vi "EvaluateBurstTriggers.vi"(8 "error in (no error)":errorcluster, 9 "data":T2, 10 "config":T1, 11 "Qbus in":refnum<class "Qbus.lvclass">) -> (0 "error out":errorcluster, 2 "config out":T1)   [LabVIEW 2017, in "BurstMode.lvlib"]
uses:
  <vilib>/addons/InsightCM/Devices/Shared/Cms/CmsBurstMode/BurstMode.lvlib
  <vilib>/addons/Qbus/Qbus.lvclass
  <vilib>/addons/InsightCM/Devices/Shared/Common/DataFlow/controls/Data.ctl
  <vilib>/addons/InsightCM/Utilities/DataAccessors/controls/wfmSGL_DVR.ctl
  <vilib>/addons/PointValueMap/controls/PointMap.ctl
  <vilib>/addons/InsightCM/Devices/Shared/Common/DataFlow/controls/Type.ctl
  <vilib>/addons/InsightCM/Devices/Shared/Cms/CmsBurstMode/controls/config.ctl
  <vilib>/addons/InsightCM/Devices/Shared/Cms/CmsBurstMode/controls/InitiateBurstMode.ctl
  <vilib>/addons/PointValueMap/PointValueMap.lvlib
  <vilib>/addons/InsightCM/Devices/Shared/Common/DataFlow/DataFlow.lvlib
panel:
  in  "force burst":bool
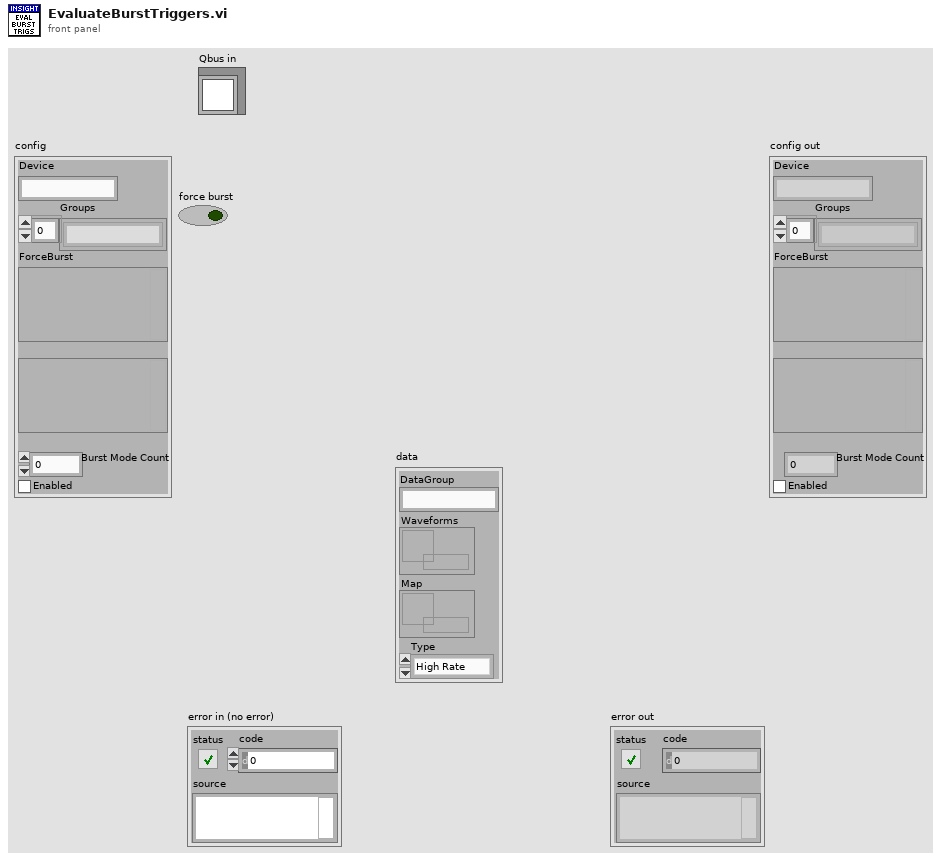
[diagram p1: front panel]
types:
  T1 = typedef "BurstMode.lvlib/config.ctl" = cluster{"Device":string, "Groups":string[], "ForceBurst":variant, "TriggerBurst":variant, "Burst Mode Count":i32, "Enabled":bool}
  T2 = typedef "DataFlow.lvlib/Data.ctl" = cluster{"DataGroup":string, "Waveforms":T3, "Map":T4, "Type":T5}
  T3 = typedef "wfmSGL_DVR.ctl" = refnum<data-value>
  T4 = typedef "PointValueMap.lvlib/PointMap.ctl" = refnum<data-value>
  T5 = typedef "DataFlow.lvlib/Type.ctl" = enum16{"High Rate", "Low Rate", "Burst Mode"}
  T6 = typedef "BurstMode.lvlib/InitiateBurstMode.ctl" = cluster{"Group":string, "Acq Reason":string}
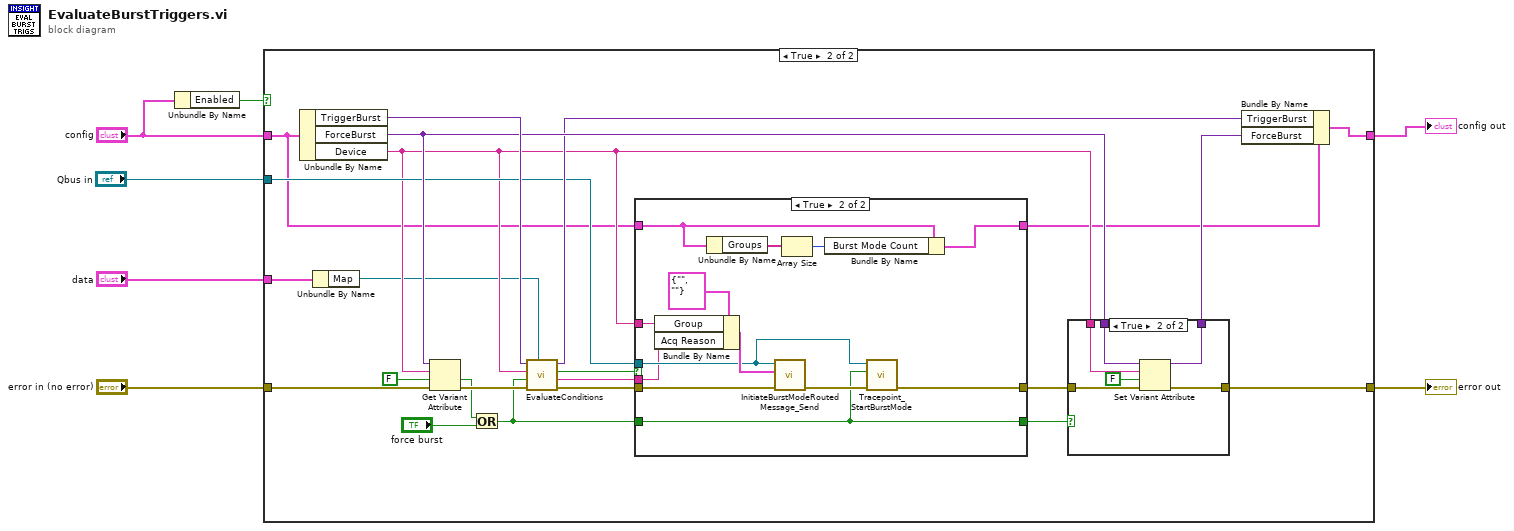
[diagram p0: block diagram]
diagram:
  n1 = Unbundle By Name("config") -> ("Enabled"=w1:bool)
  n2 = case shown="True" w1 {
    tunnel: [w8 w32] -> w7
    tunnel: "data" -> [_ w30]
    tunnel: "error in (no error)" -> [w8 w29]
    tunnel: [w9 w21] -> w4
    tunnel: "Qbus in" -> [_ w20]
    tunnel: "config" -> [w9 w13]
    frame False {
    }
    frame True {
      n3 = Unbundle By Name(w13) -> ("TriggerBurst"=w26:variant, "ForceBurst"=w25:variant, "Device"=w19:string)
      n4 = Unbundle By Name(w30) -> ("Map"=w10:T4)
      n5 = Get Variant Attribute(Variant=w25, name=w19, default value (empty Variant)=FALSE ("force trigger"), error in=w29) -> (value=w18:bool, error out=w27:errorcluster)  [unwired: 2 out]
      n6 = Or(x=w18, y="force burst") -> (x .or. y?=w16:bool)
      n7 = call <vilib>:"EvaluateConditions.vi"("map"=w10, "error in"=w27, "force burst"=w16, "device"=w19, "burst mode trigger"=w26) -> ("error out"=w23:errorcluster, "reason"=w11:string, "burst"=w14:bool, "burst mode trigger"=w22:variant)  [unwired: 3 in]
      n8 = case shown="True" w14 {
        tunnel: w23 -> [w35 w48]
        tunnel: [w35 w37] -> w31
        tunnel: w20 -> [_ w43]
        tunnel: w19 -> [_ w45]
        tunnel: [w34 w42] -> w15
        tunnel: w16 -> [w34 w42]
        tunnel: w13 -> [w33 w40]
        tunnel: [w33 w41] -> w12
        tunnel: w11 -> [_ w36]
        frame False {
        }
        frame True {
          n9 = Bundle By Name(cluster=T6 {"Group"="", "Acq Reason"=""} ("InitiateBurstMode"), "Group"=w45, "Acq Reason"=w36) -> (w46:T6)
          n10 = Unbundle By Name(w40) -> ("Groups"=w39:string[])
          n11 = call <vilib>:"InitiateBurstModeRoutedMessage_Send.vi"("error in (no error)"=w48, "InitiateBurstMode"=w46, "Qbus in"=w43) -> ("error out"=w44:errorcluster)  [unwired: 7 in, 1 out]
          n12 = Array Size(array=w39) -> (size(s)=w38:i32)
          n13 = Bundle By Name(cluster=w40, "Burst Mode Count"=w38) -> (w41:T1)
          n14 = call <vilib>:"Tracepoint_StartBurstMode.vi"("error in (no error)"=w44, "ForceBurst"=w42, "Qbus"=w43) -> ("error out"=w37:errorcluster)  [unwired: 8 in]
        }
      }
      n15 = case shown="True" w15 {
        tunnel: [w49 w56] -> w24
        tunnel: [w50 w55] -> w32
        tunnel: w25 -> [w49 w54]
        tunnel: w31 -> [w50 w53]
        tunnel: w19 -> [_ w52]
        frame False {
        }
        frame True {
          n16 = Set Variant Attribute(Variant=w54, name=w52, value=FALSE, error in=w53) -> (Variant out=w56:variant, error out=w55:errorcluster)  [unwired: 1 out]
        }
      }
      n17 = Bundle By Name(cluster=w12, "TriggerBurst"=w22, "ForceBurst"=w24) -> (w21:T1)
    }
  }
  "error out" <- w7
  "config out" <- w4
